vi "main.vi"() -> ()   [LabVIEW 2014]
uses:
  <vilib>/MakerHub/LINX/Public/Utilities/Open Local.vi
  <vilib>/MakerHub/LINX/LMH-LINX.lvlib
panel:
  in  "Sequence array":i8[](array[numeric])
  in  "Melody array":i32[][](array[numeric])
  in  "stop":bool
  out "Indicators [GYBWR]":refnum<vi>[](array[refnum])
  in  "Level":i32=3
  out "Red":bool
  out "Blue":bool
  out "Green":bool
  out "White":bool
  out "Yellow":bool
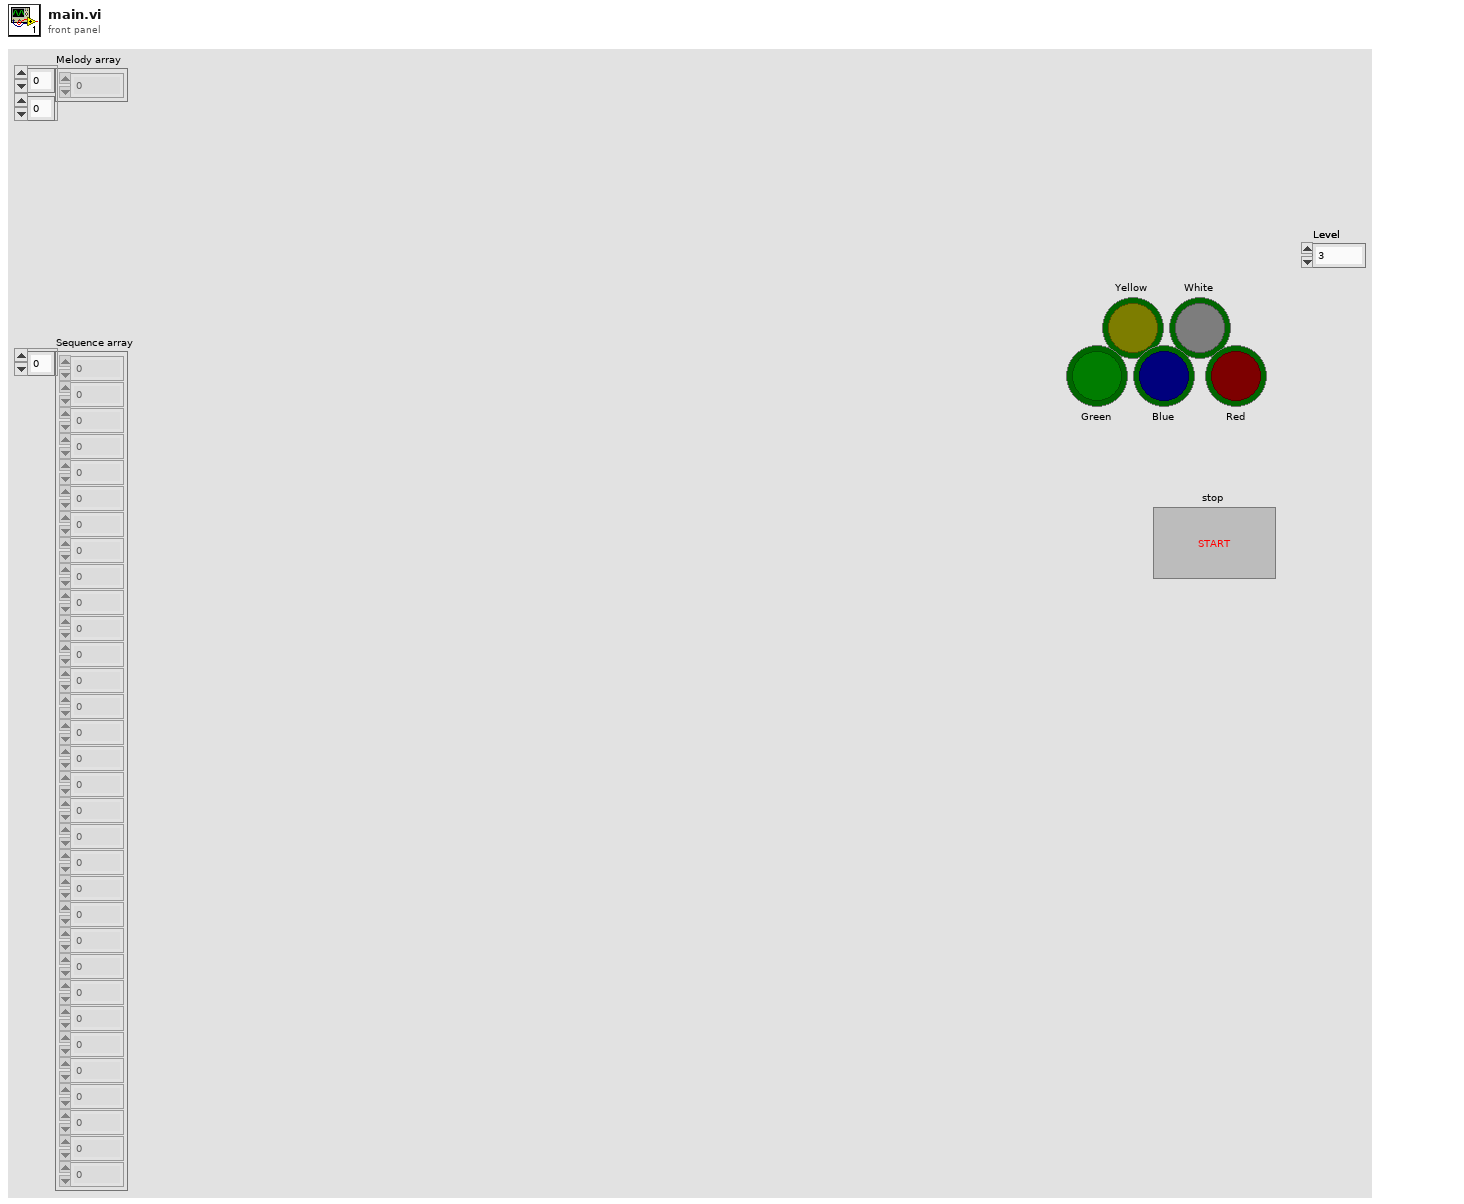
[diagram p1: front panel]
types:
  T1 = enum16{"Prepare", "Wait for start", "Lock input", "Show tones", "Generate and play sequence", "Validate input"}
  T2 = typedef "LMH-LINX.lvlib/LINX Ref.ctl" = cluster{"IO":T3, "Interface":T4, "LINX Device Config":T5}
  T3 = typedef "LMH-LINX.lvlib/Platform.ctl" = enum16{"Remote", "Local"}
  T4 = typedef "LMH-LINX.lvlib/Interface.ctl" = enum16{"Serial", "TCP"}
  T5 = typedef "LMH-LINX.lvlib/Device.lvlib/LINX Device Config.ctl" = cluster{"Interface":T4, "COM Port":refnum<visa-resource-name>, "TCP Configuration":T6, "Device Family":u8, "Device ID":u8, "Device Name":string, "TCP Ref":refnum<k5>, "Channels":T7}
  T6 = typedef "LMH-LINX.lvlib/Device.lvlib/TCP Config.ctl" = cluster{"IP Address":string, "Port":u16}
  T7 = typedef "LMH-LINX.lvlib/Channels.ctl" = cluster{"DI":u8[], "DO":u8[], "AI":u8[], "AO":u8[], "PWM":u8[], "QE":u8[], "UART":u8[], "I2C 2":u8[], "SPI":u8[], "CAN":u8[], "Servo":u8[], "AI Ref (V)":dbl, "AI Resolution (Bits)":u8, "AO Ref (V)":dbl, "AO Resolution (Bits)":u8}
  T8 = enum8{"Enabled", "Disabled", "Disabled and Grayed Out"}
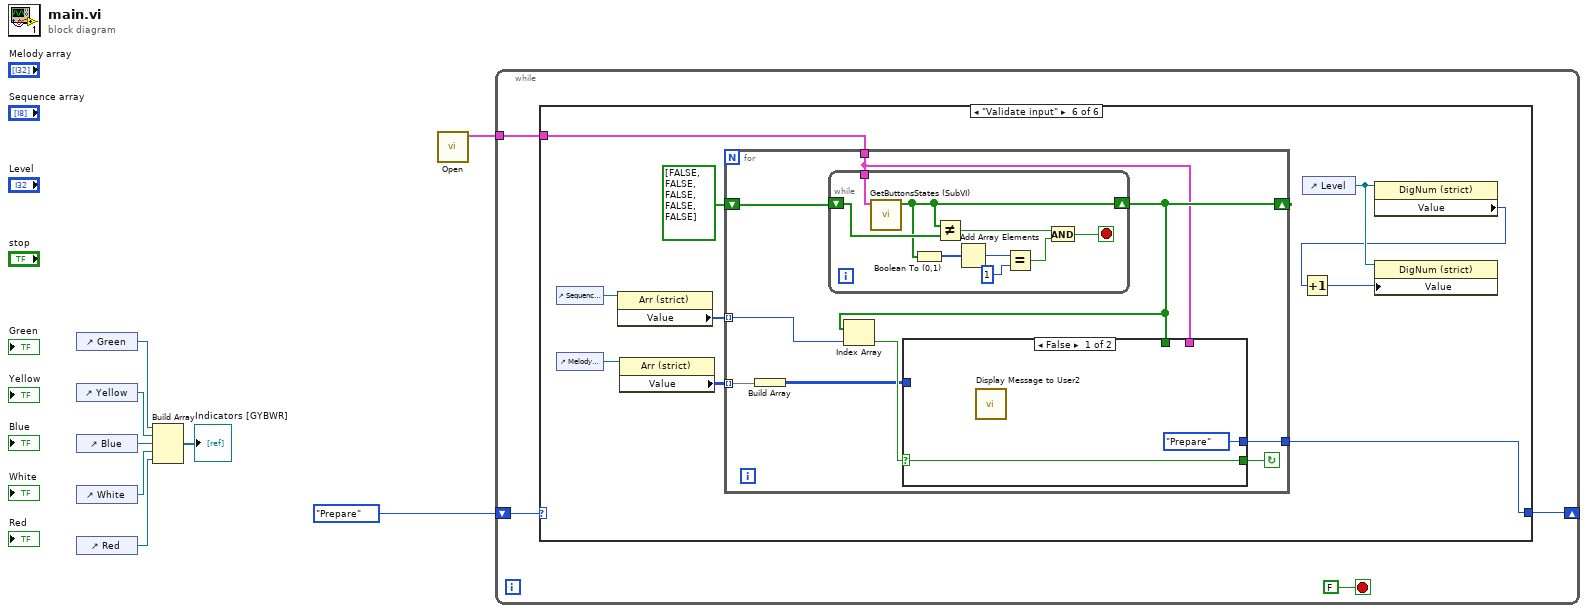
[diagram p0: block diagram]
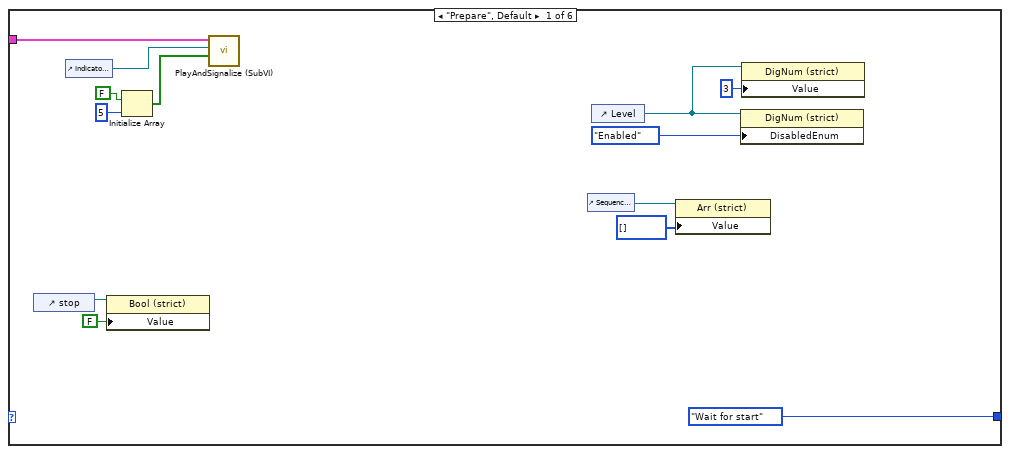
[diagram p2: hidden frame]
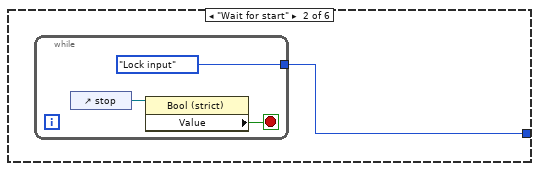
[diagram p3: hidden frame]
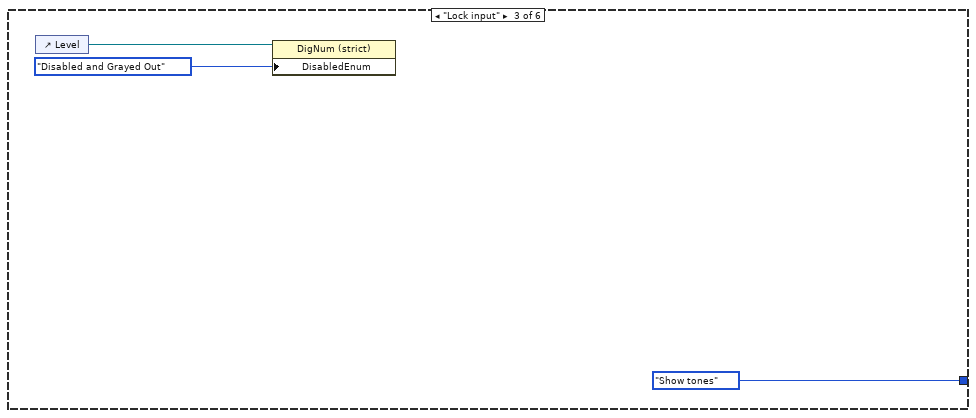
[diagram p4: hidden frame]
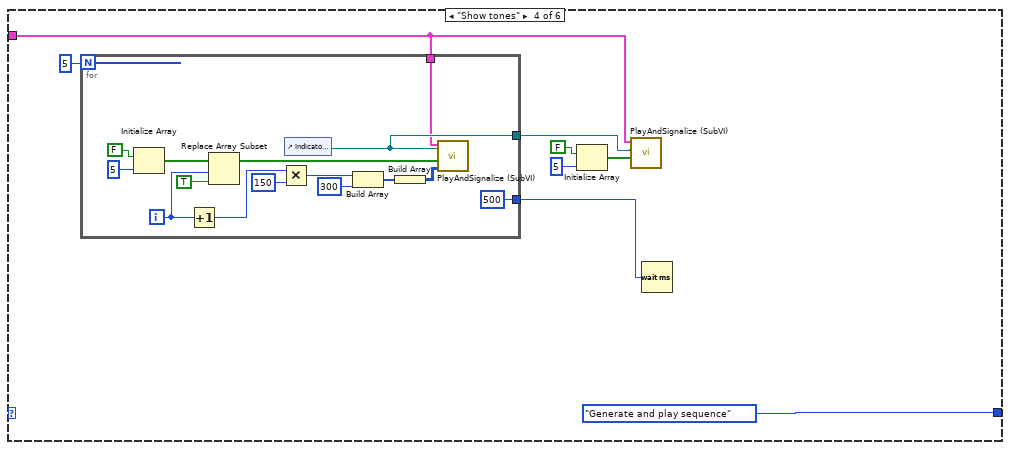
[diagram p5: hidden frame]
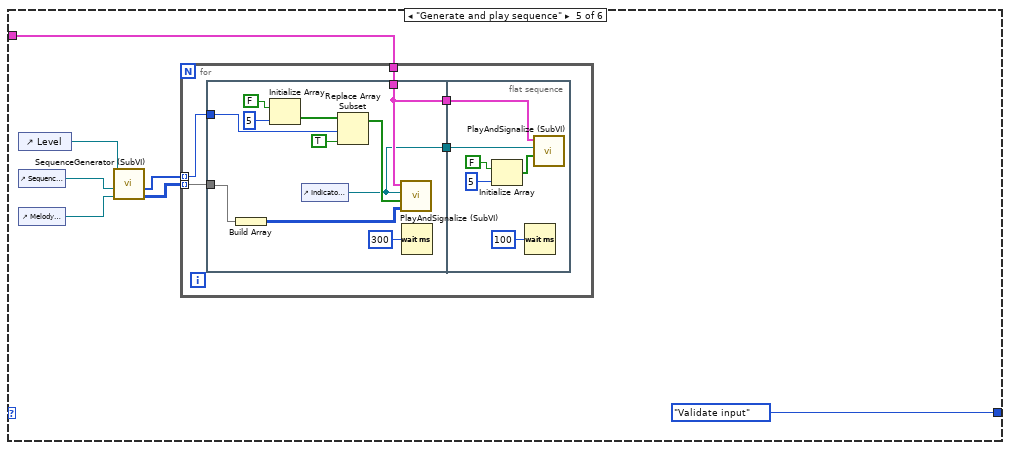
[diagram p6: hidden frame]
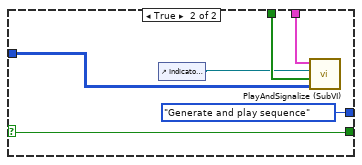
[diagram p7: hidden frame]
diagram:
  n1 = control-ref of="Green"() -> (w3:refnum<vi>)
  n2 = control-ref of="Yellow"() -> (w6:refnum<vi>)
  n3 = control-ref of="Blue"() -> (w5:refnum<vi>)
  n4 = control-ref of="White"() -> (w7:refnum<vi>)
  n5 = control-ref of="Red"() -> (w8:refnum<vi>)
  n6 = Build Array(w3, w6, w5, w7, w8) -> (→"Indicators [GYBWR]":refnum<vi>[])
  n7 = call-poly <vilib>:"Open.vi"() -> ("LINX Resource"=w1:T2)  [unwired: 9 in, 2 out]
  n8 = while {
    shift-right: [w11] -> _
    shift-left: T1."Prepare" -> [w12]
    tunnel: w1 -> [w10]
    stop <- FALSE stop-if-true
    n9 = case shown="\"Validate input\"" w12 {
      tunnel: [T1."Wait for start" w26 T1."Show tones" T1."Generate and play sequence" T1."Validate input" w85] -> w11
      tunnel: w10 -> [w21 _ _ w33 w60 w93]
      frame "Prepare", Default {
        n10 = control-ref of="stop"() -> (w18:refnum<vi>)
        n11 = control-ref of="Indicators [GYBWR]"() -> (w20:refnum<vi>)
        n12 = property class="Bool (strict)"(reference=w18, "Value"=FALSE) -> ()  [unwired: 1 in, 2 out]
        n13 = Initialize Array(FALSE, 5 ("dimension size")) -> (w24:bool[])
        n14 = call "PlayAndSignalize (SubVI).vi"("State [GYBWR]"=w24, "Indicators [GYBWR]"=w20, "LINX Resource"=w21) -> ()  [unwired: 9 in]
        n15 = control-ref of="Sequence array"() -> (w14:refnum<vi>)
        n16 = control-ref of="Level"() -> (w16:refnum<vi>)
        n17 = property class="Arr (strict)"(reference=w14, "Value"=i8[] []) -> ()  [unwired: 1 in, 2 out]
        n18 = property class="DigNum (strict)"(reference=w16, "DisabledEnum"=T8."Enabled" ("Disabled")) -> ()  [unwired: 1 in, 2 out]
        n19 = property class="DigNum (strict)"(reference=w16, "Value"=3) -> ()  [unwired: 1 in, 2 out]
      }
      frame "Wait for start" {
        n20 = while {
          tunnel: [T1."Lock input"] -> w26
          stop <- w29 stop-if-true
          n21 = control-ref of="stop"() -> (w28:refnum<vi>)
          n22 = property class="Bool (strict)"(reference=w28) -> ("Value"=w29:bool)  [unwired: 1 in, 2 out]
        }
      }
      frame "Lock input" {
        n23 = control-ref of="Level"() -> (w31:refnum<vi>)
        n24 = property class="DigNum (strict)"(reference=w31, "DisabledEnum"=T8."Disabled and Grayed Out" ("Disabled")) -> ()  [unwired: 1 in, 2 out]
      }
      frame "Show tones" {
        n25 = for {
          N: 5 -> [_]
          tunnel: [w42] -> w36
          tunnel: [500] -> w35
          tunnel: w33 -> [w41]
          i -> [w45]
          n26 = Initialize Array(FALSE, 5 ("dimension size")) -> (w54:bool[])
          n27 = Increment(x=w45) -> (x+1=w44:i32)
          n28 = Replace Array Subset(array=w54, new element=TRUE ("new element/subarray"), index=w45) -> (w46:bool[])
          n29 = Multiply(x=w44, y=150) -> (x*y=w50:i32)
          n30 = control-ref of="Indicators [GYBWR]"() -> (w42:refnum<vi>)
          n31 = Build Array(w50, 300 ("element")) -> (w48:i32[])
          n32 = Build Array(w48) -> (w47:i32[][])
          n33 = call "PlayAndSignalize (SubVI).vi"("Tone (Frequency:Duration)"=w47, "State [GYBWR]"=w46, "Indicators [GYBWR]"=w42, "LINX Resource"=w41) -> ()  [unwired: 8 in]
        }
        n34 = Initialize Array(FALSE, 5 ("dimension size")) -> (w37:bool[])
        n35 = call "PlayAndSignalize (SubVI).vi"("State [GYBWR]"=w37, "Indicators [GYBWR]"=w36, "LINX Resource"=w33) -> ()  [unwired: 9 in]
        n36 = Wait (ms)(milliseconds to wait=w35) -> ()  [unwired: 1 out]
      }
      frame "Generate and play sequence" {
        n37 = control-ref of="Level"() -> (w62:refnum<vi>)
        n38 = control-ref of="Sequence array"() -> (w57:refnum<vi>)
        n39 = control-ref of="Melody array"() -> (w56:refnum<vi>)
        n40 = call "SequenceGenerator (SubVI).vi"("Melody array (in)"=w56, "Sequence array (in)"=w57, "Elements number"=w62) -> ("Melody array (out)"=w58:i32[][], "Sequence array (out)"=w59:i8[])  [unwired: 7 in]
        n41 = for {
          tunnel: w59 -> [w66] mode=indexing
          tunnel: w58 -> [w67] mode=indexing
          tunnel: w60 -> [w65]
          n42 = flat-sequence {
            tunnel: w67 -> [w78]
            tunnel: w66 -> [w71]
            tunnel: w65 -> [w70]
            tunnel: [w70] -> w64
            tunnel: [w69] -> w63
            tunnel: w64 -> [w81]
            tunnel: w63 -> [w80]
            frame #0 {
              n43 = Build Array(w78) -> (w72:i32[][])
              n44 = Initialize Array(FALSE, 5 ("dimension size")) -> (w75:bool[])
              n45 = control-ref of="Indicators [GYBWR]"() -> (w69:refnum<vi>)
              n46 = Replace Array Subset(array=w75, new element=TRUE ("new element/subarray"), index=w71) -> (w73:bool[])
              n47 = call "PlayAndSignalize (SubVI).vi"("Tone (Frequency:Duration)"=w72, "State [GYBWR]"=w73, "Indicators [GYBWR]"=w69, "LINX Resource"=w70) -> ()  [unwired: 8 in]
              n48 = Wait (ms)(milliseconds to wait=u32 300) -> ()  [unwired: 1 out]
            }
            frame #1 {
              n49 = Initialize Array(FALSE, 5 ("dimension size")) -> (w82:bool[])
              n50 = Wait (ms)(milliseconds to wait=u32 100) -> ()  [unwired: 1 out]
              n51 = call "PlayAndSignalize (SubVI).vi"("State [GYBWR]"=w82, "Indicators [GYBWR]"=w80, "LINX Resource"=w81) -> ()  [unwired: 9 in]
            }
          }
        }
      }
      frame "Validate input" {
        n52 = control-ref of="Sequence array"() -> (w90:refnum<vi>)
        n53 = control-ref of="Melody array"() -> (w89:refnum<vi>)
        n54 = property class="Arr (strict)"(reference=w90) -> ("Value"=w91:i8[])  [unwired: 1 in, 2 out]
        n55 = property class="Arr (strict)"(reference=w89) -> ("Value"=w92:i32[][])  [unwired: 1 in, 2 out]
        n56 = for {
          tunnel: w93 -> [w98]
          shift-right: [w101] -> _
          shift-left: bool[] [FALSE, FALSE, FALSE, FALSE, FALSE] ("Buttons [GYBWR]") -> [w103]
          tunnel: w92 -> [w97] mode=indexing
          tunnel: w91 -> [w96] mode=indexing
          tunnel: [w95] -> w85
          stop <- w99 continue-if-true
          n57 = Build Array(w97) -> (w100:i32[][])
          n58 = while {
            tunnel: w98 -> [w120]
            shift-right: [w117] -> w101
            shift-left: w103 -> [w119]
            stop <- w112 stop-if-true
            n59 = call "GetButtonsStates (SubVI).vi"("LINX Resource"=w120) -> ("Buttons [GYBWR]"=w117:bool[])  [unwired: 10 in]
            n60 = Boolean To (0,1)(Boolean=w117) -> (0, 1=w118:i16[])
            n61 = Not Equal?(x=w117, y=w119) -> (x != y?=w116:bool)
            n62 = Add Array Elements(numeric array=w118) -> (sum=w114:i16)
            n63 = Equal?(x=w114, y=i16 1) -> (x = y?=w113:bool)
            n64 = And(x=w116, y=w113) -> (x .and. y?=w112:bool)
          }
          n65 = Index Array(array=w101, index=w96) -> (element=w102:bool)
          n66 = case shown="False" w102 {
            selector: w102 -> [w105 w108]
            tunnel: w98 -> [_ w111]
            tunnel: w101 -> [_ w110]
            tunnel: w100 -> [_ w109]
            tunnel: [w105 w108] -> w99
            tunnel: [T1."Prepare" T1."Generate and play sequence"] -> w95
            frame False {
              n67 = call "Display Message to User2"() -> ()  [unwired: 10 in, 2 out]
            }
            frame True {
              n68 = control-ref of="Indicators [GYBWR]"() -> (w107:refnum<vi>)
              n69 = call "PlayAndSignalize (SubVI).vi"("Tone (Frequency:Duration)"=w109, "State [GYBWR]"=w110, "Indicators [GYBWR]"=w107, "LINX Resource"=w111) -> ()  [unwired: 8 in]
            }
          }
        }
        n70 = control-ref of="Level"() -> (w88:refnum<vi>)
        n71 = property class="DigNum (strict)"(reference=w88) -> ("Value"=w86:i32)  [unwired: 1 in, 2 out]
        n72 = Increment(x=w86) -> (x+1=w87:i32)
        n73 = property class="DigNum (strict)"(reference=w88, "Value"=w87) -> ()  [unwired: 1 in, 2 out]
      }
    }
  }
